vi "GetSubversionRevision.vi"(11 "File Path Control":path caption="File Path Control (leave blank to use Constants_Global value of EnFlo SW Folder)") -> (0 "This Folder's Last Changed Date":string, 1 "This Folder's Last Revision":string, 2 "LocalModifications":string, 3 "OverallRevision":string, 4 "standard error":string, 5 "standard output":string)   [LabVIEW 2011]
doc: "This VI uses the system's installed svn (subversion) software to return the revision number of the selected folder. Leaving the selected folder blank will use the global value of \"EnFlo SW Folder\".\nThe \"Overall Revision\" is the highest revision number in the entire hierarchy, recursing upwards as well as downwards- in other words, the revision which was checked out. The \"This Folder\" data is specific to the last changes to the selected folder."
uses:
  Globals/Constants_global.vi
panel:
  out "This Folder Last Committed By":string
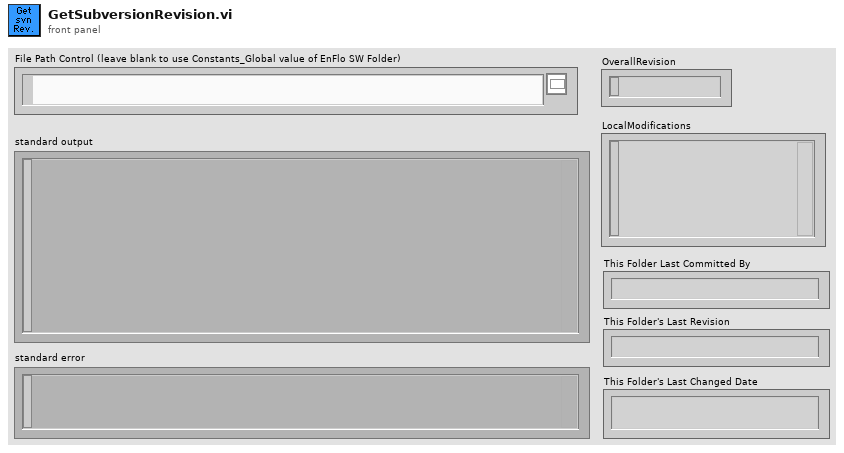
[diagram p1: front panel]
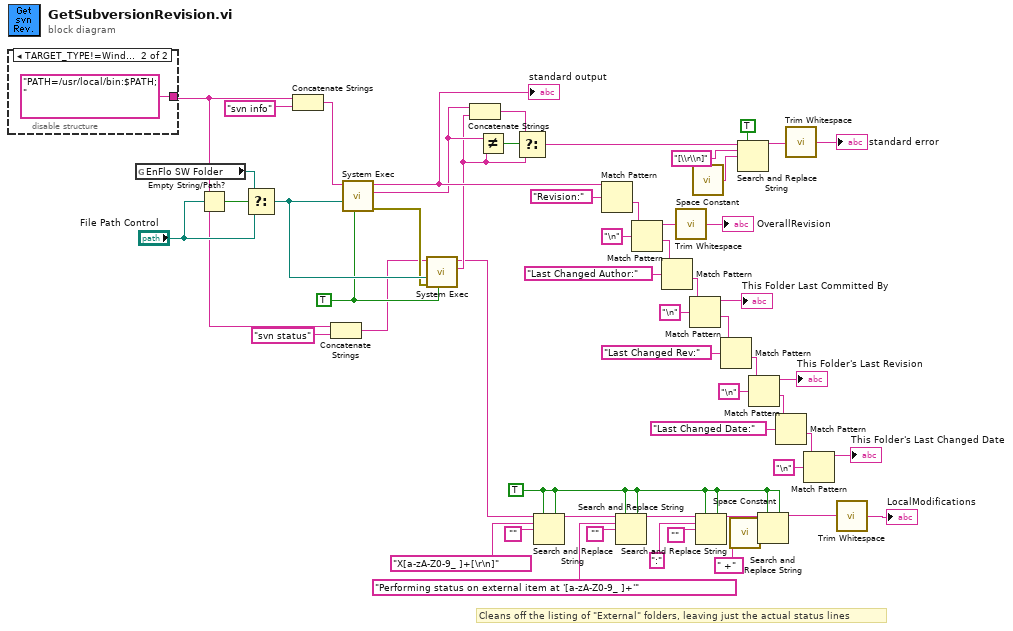
[diagram p0: block diagram]
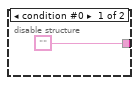
[diagram p2: hidden frame]
diagram:
  w13 = TRUE ("replace all? (F)")
  w33 = TRUE ("run minimized? (F)")
  # "Cleans off the listing of \"External\" folders, leaving just the actual status lines"
  n1 = disable-structure shown="TARGET_TYPE!=Windows" {
    disable-tunnel: ["" ("command line") "PATH=/usr/local/bin:$PATH; " ("command line")] -> w1
    frame condition #0 {
    }
    frame condition #1 (active) {
    }
  }
  n2 = global read "Constants_global.vi" "EnFlo SW Folder"() -> (w55:path)
  n3 = Empty String/Path?(string/path="File Path Control") -> (empty?=w57:bool)
  n4 = Select(t=w55, s=w57, f="File Path Control") -> (s? t:f=w34:path)
  n5 = Concatenate Strings(w1, "svn info" ("command line")) -> (w5:string)
  n6 = Concatenate Strings(w1, "svn status" ("command line")) -> (w3:string)
  n7 = call <vilib>:"System Exec.vi"("run minimized? (F)"=w33, "working directory"=w34, "command line"=w5) -> ("error out"=w32:errorcluster, "standard error"=w29:string, "standard output"=w54:string)  [unwired: 5 in, 1 out]
  "standard output" <- w54
  n8 = call <vilib>:"System Exec.vi"("run minimized? (F)"=w33, "error in (no error)"=w32, "working directory"=w34, "command line"=w3) -> ("standard error"=w26:string, "standard output"=w23:string)  [unwired: 4 in, 2 out]
  n9 = Concatenate Strings(w29, w26) -> (w27:string)
  n10 = Not Equal?(x=w29, y=w26) -> (x != y?=w28:bool)
  n11 = Select(t=w27, s=w28, f=w26) -> (s? t:f=w7:string)
  n12 = Search and Replace String(replace all?=w13, multiline?=w13, input string=w23, search string="X[a-zA-Z0-9_ ]+[\r\n]", replace string="") -> (result string=w20:string)  [unwired: 3 in, 3 out]
  n13 = Match Pattern(string=w54, regular expression="Revision:") -> (after substring=w52:string)  [unwired: 1 in, 3 out]
  n14 = Search and Replace String(replace all?=w13, multiline?=w13, input string=w20, search string="Performing status on external item at '[a-zA-Z0-9_ ]+'", replace string="") -> (result string=w18:string)  [unwired: 3 in, 3 out]
  n15 = Match Pattern(string=w52, regular expression="\n") -> (before substring=w50:string, after substring=w49:string)  [unwired: 1 in, 2 out]
  n16 = Match Pattern(string=w49, regular expression="Last Changed Author:") -> (after substring=w46:string)  [unwired: 1 in, 3 out]
  n17 = call <vilib>:"Trim Whitespace.vi"("string"=w50) -> ("trimmed string"=→"OverallRevision":string)  [unwired: 1 in]
  n18 = Match Pattern(string=w46, regular expression="\n") -> (before substring=→"This Folder Last Committed By":string, after substring=w42:string)  [unwired: 1 in, 2 out]
  n19 = call <vilib>:"Space Constant.vi"() -> ("String"=w9:string)
  n20 = Search and Replace String(replace all?=w13, multiline?=w13, input string=w18, search string=":", replace string="") -> (result string=w15:string)  [unwired: 3 in, 3 out]
  n21 = Match Pattern(string=w42, regular expression="Last Changed Rev:") -> (after substring=w44:string)  [unwired: 1 in, 3 out]
  n22 = call <vilib>:"Space Constant.vi"() -> ("String"=w11:string)
  n23 = Search and Replace String(replace all?=TRUE ("replace all? (F)"), input string=w7, search string="[\\r\\n]", replace string=w9) -> (result string=w6:string)  [unwired: 4 in, 3 out]
  n24 = Match Pattern(string=w44, regular expression="\n") -> (before substring=→"This Folder's Last Revision":string, after substring=w37:string)  [unwired: 1 in, 2 out]
  n25 = Search and Replace String(replace all?=w13, multiline?=w13, input string=w15, search string=" +", replace string=w11) -> (result string=w14:string)  [unwired: 3 in, 3 out]
  n26 = Match Pattern(string=w37, regular expression="Last Changed Date:") -> (after substring=w38:string)  [unwired: 1 in, 3 out]
  n27 = call <vilib>:"Trim Whitespace.vi"("string"=w6) -> ("trimmed string"=→"standard error":string)  [unwired: 1 in]
  n28 = Match Pattern(string=w38, regular expression="\n") -> (before substring=→"This Folder's Last Changed Date":string)  [unwired: 1 in, 3 out]
  n29 = call <vilib>:"Trim Whitespace.vi"("string"=w14) -> ("trimmed string"=→"LocalModifications":string)  [unwired: 1 in]
